vi "ChipDateDirectory.vi"(2 "time stamp":timestamp, 3 "chipNumber":string) -> (0 "path":path, 1 "justDate":string)   [LabVIEW 2014]
uses:
  Global/Global 1.vi
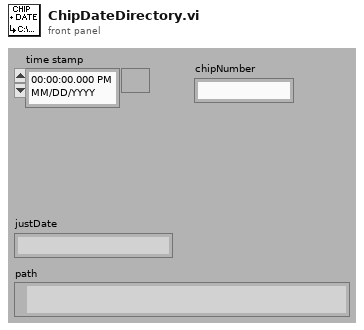
[diagram p1: front panel]
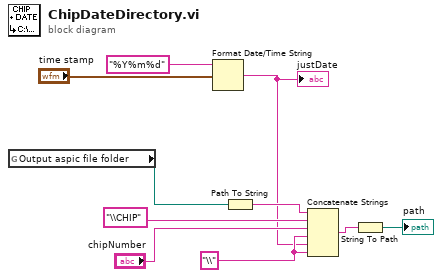
[diagram p0: block diagram]
diagram:
  w10 = "\\"
  n1 = global read "Global 1.vi" "Output aspic file folder"() -> (w1:path)
  n2 = Format Date/Time String(time format string (%c)="%Y%m%d", seconds (now)="time stamp") -> (date/time string=w4:string)  [unwired: 1 in]
  "justDate" <- w4
  n3 = Path To String(path=w1) -> (string=w8:string)
  n4 = Concatenate Strings(w8, "\\CHIP", "chipNumber", w10, w4, w10) -> (w5:string)
  n5 = String To Path(string=w5) -> (path=→"path":path)
